vi "Sched select.vi"() -> (0 "Close":bool, 1 "Load":bool, 3 "selected sched":string)   [LabVIEW 2023]
uses:
  Sched select.ctl
panel:
  in  "stop":bool
  in  "Schedules":T1
  out "SchedNames":string[](array[string])
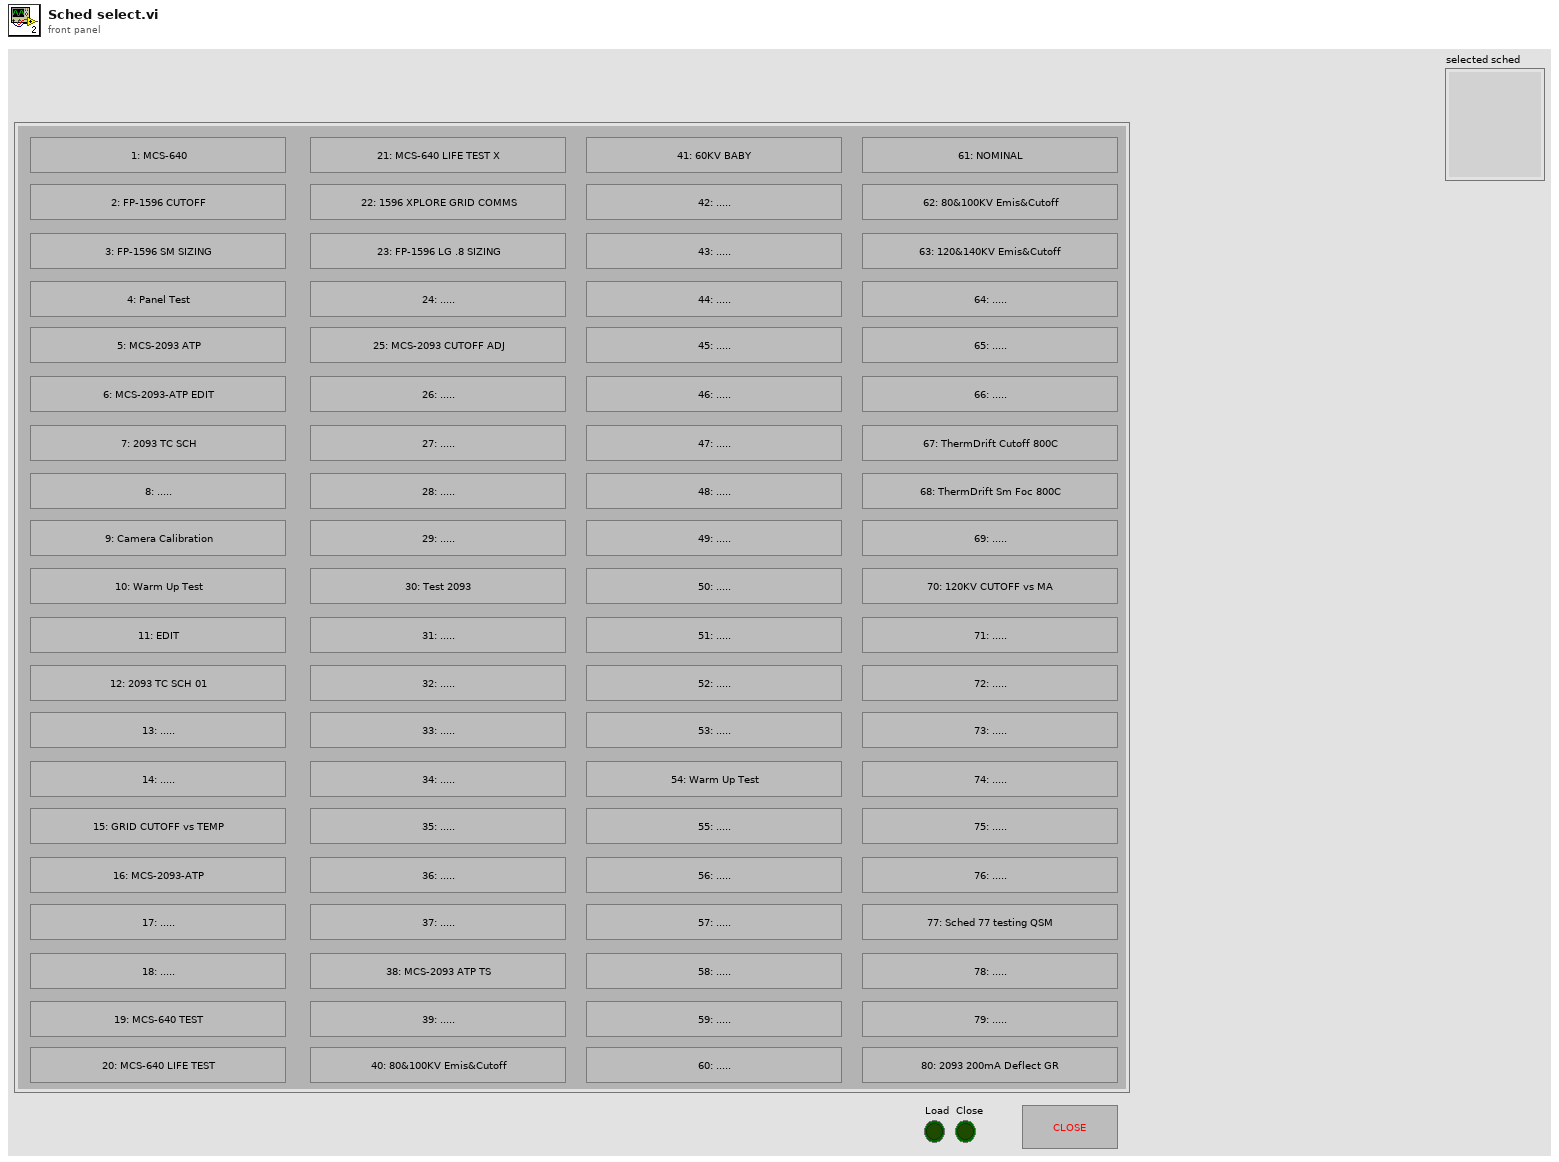
[diagram p1: front panel]
types:
  T1 = typedef "Sched select.ctl" = cluster{"OK Button 1":bool, "OK Button 2":bool, "OK Button 3":bool, "OK Button 4":bool, "OK Button 5":bool, "OK Button 6":bool, "OK Button 7":bool, "OK Button 8":bool, "OK Button 9":bool, "OK Button 10":bool, "OK Button 11":bool, "OK Button 12":bool, "OK Button 13":bool, "OK Button 14":bool, "OK Button 15":bool, "OK Button 16":bool, "OK Button 17":bool, "OK Button 18":bool, "OK Button 19":bool, "OK Button 20":bool, "OK Button 21":bool, "OK Button 22":bool, "OK Button 23":bool, "OK Button 24":bool, "OK Button 25":bool, "OK Button 26":bool, "OK Button 27":bool, "OK Button 28":bool, "OK Button 29":bool, "OK Button 30":bool, "OK Button 31":bool, "OK Button 32":bool, "OK Button 33":bool, "OK Button 34":bool, "OK Button 35":bool, "OK Button 36":bool, "OK Button 37":bool, "OK Button 38":bool, "OK Button 39":bool, "OK Button 40":bool, "OK Button 41":bool, "OK Button 42":bool, "OK Button 43":bool, "OK Button 44":bool, "OK Button 45":bool, "OK Button 46":bool, "OK Button 47":bool, "OK Button 48":bool, "OK Button 49":bool, "OK Button 50":bool, "OK Button 51":bool, "OK Button 52":bool, "OK Button 53":bool, "OK Button 54":bool, "OK Button 55":bool, "OK Button 56":bool, "OK Button 57":bool, "OK Button 58":bool, "OK Button 59":bool, "OK Button 60":bool, "OK Button 61":bool, "OK Button 62":bool, "OK Button 63":bool, "OK Button 64":bool, "OK Button 65":bool, "OK Button 66":bool, "OK Button 67":bool, "OK Button 68":bool, "OK Button 69":bool, "OK Button 70":bool, "OK Button 71":bool, "OK Button 72":bool, "OK Button 73":bool, "OK Button 74":bool, "OK Button 75":bool, "OK Button 76":bool, "OK Button 77":bool, "OK Button 78":bool, "OK Button 79":bool, "OK Button 80":bool}
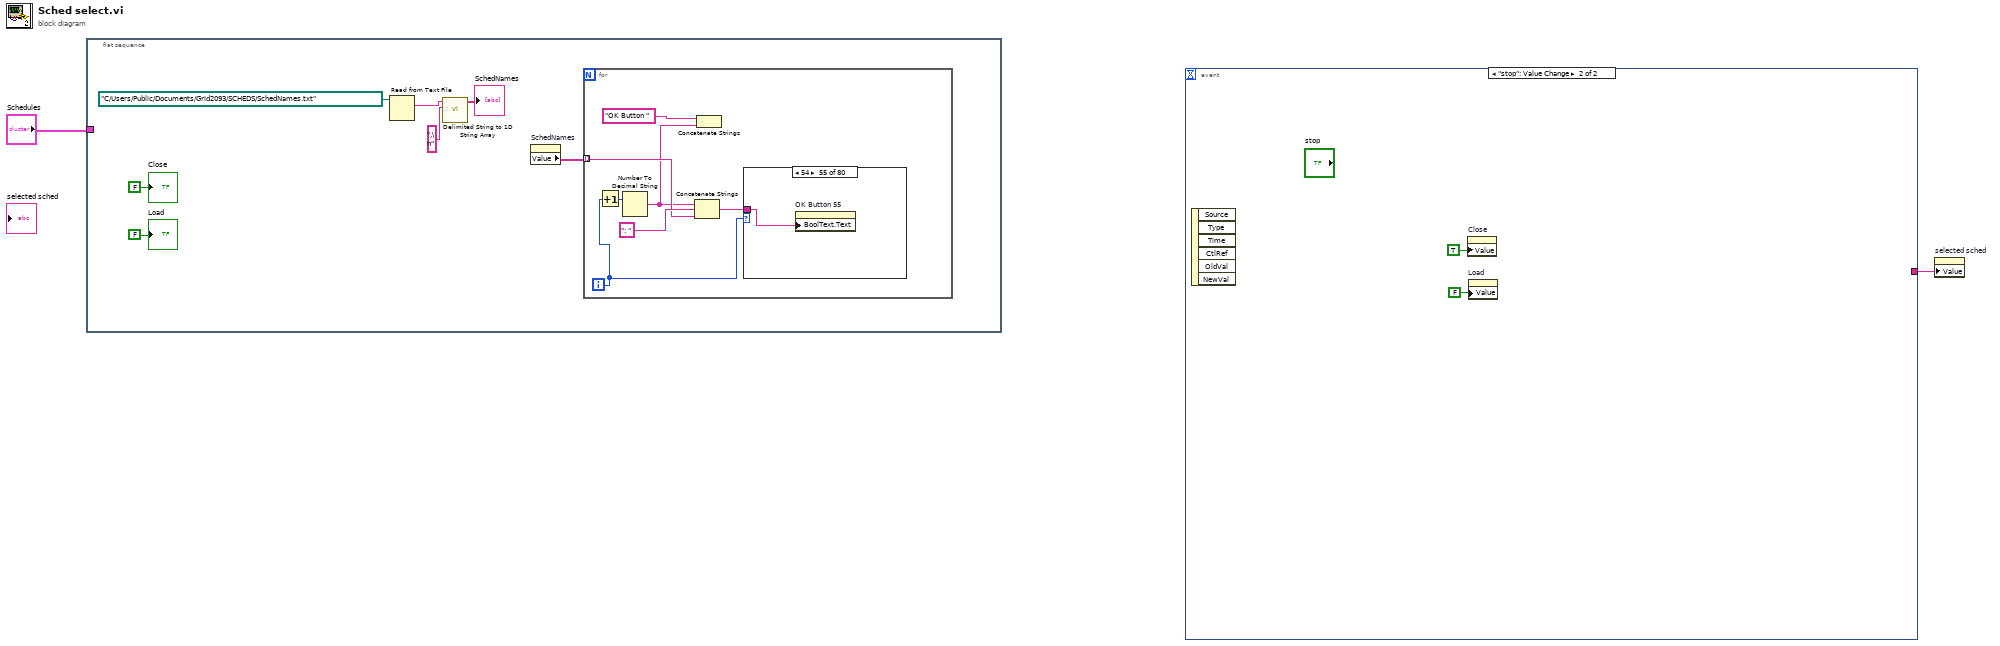
[diagram p0: block diagram]
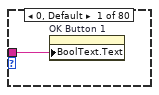
[diagram p2: hidden frame]
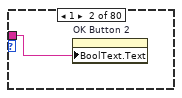
[diagram p3: hidden frame]
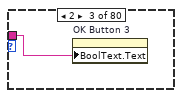
[diagram p4: hidden frame]
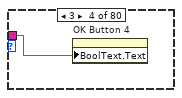
[diagram p5: hidden frame]
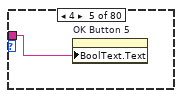
[diagram p6: hidden frame]
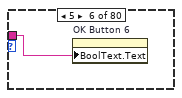
[diagram p7: hidden frame]
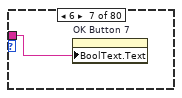
[diagram p8: hidden frame]
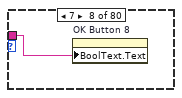
[diagram p9: hidden frame]
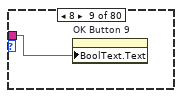
[diagram p10: hidden frame]
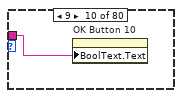
[diagram p11: hidden frame]
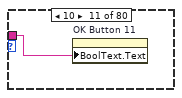
[diagram p12: hidden frame]
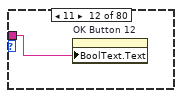
[diagram p13: hidden frame]
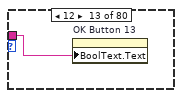
[diagram p14: hidden frame]
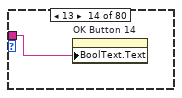
[diagram p15: hidden frame]
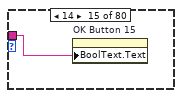
[diagram p16: hidden frame]
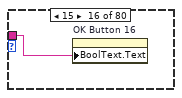
[diagram p17: hidden frame]
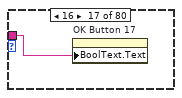
[diagram p18: hidden frame]
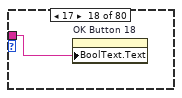
[diagram p19: hidden frame]
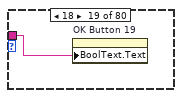
[diagram p20: hidden frame]
diagram:
  n1 = flat-sequence {
    tunnel: "Schedules" -> [_]
    frame #0 {
      n2 = Read from Text File(file (use dialog)=path "C:/Users/Public/Documents/Grid2093/SCHEDS/SchedNames.txt") -> (text=w9:string)  [unwired: 3 in, 3 out]
      n3 = call <vilib>:"Delimited String to 1D String Array.vi"("delimiter"=",\n", "delimited string"=w9) -> ("string array"=→"SchedNames":string[])  [unwired: 9 in]
      n4 = property on="SchedNames" class="Arr (strict)"() -> ("Value"=w6:string[])  [unwired: 2 in, 2 out]
      n5 = for {
        tunnel: w6 -> [w15] mode=indexing
        i -> [w11]
        n6 = Increment(x=w11) -> (x+1=w12:i32)
        n7 = Number To Decimal String(number=w12) -> (decimal integer string=w13:string)  [unwired: 1 in]
        n8 = Concatenate Strings(w13, ": " ("string"), w15) -> (w10:string)
        n9 = Concatenate Strings("OK Button ", w13) -> ()  [unwired: 1 out]
        n10 = case shown="54" w11 {
          tunnel: w10 -> [w17 w18 w19 w20 w21 w22 w23 w24 w25 w26 w27 w28 w29 w30 w31 w32 w33 w34 w35 w36 w37 w38 w39 w40 w41 w42 w43 w44 w45 w46 w47 w48 w49 w50 w51 w52 w53 w54 w55 w56 w57 w58 w59 w60 w61 w62 w63 w64 w65 w66 w67 w68 w69 w70 w71 w72 w73 w74 w75 w76 w77 w78 w79 w80 w81 w82 w83 w84 w85 w86 w87 w88 w89 w90 w91 w92 w93 w94 w95 w96]
          frame 0, Default {
            n11 = property on="OK Button 1" class="Bool (strict)"("BoolText.Text"=w17) -> ()  [unwired: 2 in, 2 out]
          }
          frame 1 {
            n12 = property on="OK Button 2" class="Bool (strict)"("BoolText.Text"=w18) -> ()  [unwired: 2 in, 2 out]
          }
          frame 2 {
            n13 = property on="OK Button 3" class="Bool (strict)"("BoolText.Text"=w19) -> ()  [unwired: 2 in, 2 out]
          }
          frame 3 {
            n14 = property on="OK Button 4" class="Bool (strict)"("BoolText.Text"=w20) -> ()  [unwired: 2 in, 2 out]
          }
          frame 4 {
            n15 = property on="OK Button 5" class="Bool (strict)"("BoolText.Text"=w21) -> ()  [unwired: 2 in, 2 out]
          }
          frame 5 {
            n16 = property on="OK Button 6" class="Bool (strict)"("BoolText.Text"=w22) -> ()  [unwired: 2 in, 2 out]
          }
          frame 6 {
            n17 = property on="OK Button 7" class="Bool (strict)"("BoolText.Text"=w23) -> ()  [unwired: 2 in, 2 out]
          }
          frame 7 {
            n18 = property on="OK Button 8" class="Bool (strict)"("BoolText.Text"=w24) -> ()  [unwired: 2 in, 2 out]
          }
          frame 8 {
            n19 = property on="OK Button 9" class="Bool (strict)"("BoolText.Text"=w25) -> ()  [unwired: 2 in, 2 out]
          }
          frame 9 {
            n20 = property on="OK Button 10" class="Bool (strict)"("BoolText.Text"=w26) -> ()  [unwired: 2 in, 2 out]
          }
          frame 10 {
            n21 = property on="OK Button 11" class="Bool (strict)"("BoolText.Text"=w27) -> ()  [unwired: 2 in, 2 out]
          }
          frame 11 {
            n22 = property on="OK Button 12" class="Bool (strict)"("BoolText.Text"=w28) -> ()  [unwired: 2 in, 2 out]
          }
          frame 12 {
            n23 = property on="OK Button 13" class="Bool (strict)"("BoolText.Text"=w29) -> ()  [unwired: 2 in, 2 out]
          }
          frame 13 {
            n24 = property on="OK Button 14" class="Bool (strict)"("BoolText.Text"=w30) -> ()  [unwired: 2 in, 2 out]
          }
          frame 14 {
            n25 = property on="OK Button 15" class="Bool (strict)"("BoolText.Text"=w31) -> ()  [unwired: 2 in, 2 out]
          }
          frame 15 {
            n26 = property on="OK Button 16" class="Bool (strict)"("BoolText.Text"=w32) -> ()  [unwired: 2 in, 2 out]
          }
          frame 16 {
            n27 = property on="OK Button 17" class="Bool (strict)"("BoolText.Text"=w33) -> ()  [unwired: 2 in, 2 out]
          }
          frame 17 {
            n28 = property on="OK Button 18" class="Bool (strict)"("BoolText.Text"=w34) -> ()  [unwired: 2 in, 2 out]
          }
          frame 18 {
            n29 = property on="OK Button 19" class="Bool (strict)"("BoolText.Text"=w35) -> ()  [unwired: 2 in, 2 out]
          }
          frame 19 {
            n30 = property on="OK Button 20" class="Bool (strict)"("BoolText.Text"=w36) -> ()  [unwired: 2 in, 2 out]
          }
          frame 20 {
            n31 = property on="OK Button 21" class="Bool (strict)"("BoolText.Text"=w37) -> ()  [unwired: 2 in, 2 out]
          }
          frame 21 {
            n32 = property on="OK Button 22" class="Bool (strict)"("BoolText.Text"=w38) -> ()  [unwired: 2 in, 2 out]
          }
          frame 22 {
            n33 = property on="OK Button 23" class="Bool (strict)"("BoolText.Text"=w39) -> ()  [unwired: 2 in, 2 out]
          }
          frame 23 {
            n34 = property on="OK Button 24" class="Bool (strict)"("BoolText.Text"=w40) -> ()  [unwired: 2 in, 2 out]
          }
          frame 24 {
            n35 = property on="OK Button 25" class="Bool (strict)"("BoolText.Text"=w41) -> ()  [unwired: 2 in, 2 out]
          }
          frame 25 {
            n36 = property on="OK Button 26" class="Bool (strict)"("BoolText.Text"=w42) -> ()  [unwired: 2 in, 2 out]
          }
          frame 26 {
            n37 = property on="OK Button 27" class="Bool (strict)"("BoolText.Text"=w43) -> ()  [unwired: 2 in, 2 out]
          }
          frame 27 {
            n38 = property on="OK Button 28" class="Bool (strict)"("BoolText.Text"=w44) -> ()  [unwired: 2 in, 2 out]
          }
          frame 28 {
            n39 = property on="OK Button 29" class="Bool (strict)"("BoolText.Text"=w45) -> ()  [unwired: 2 in, 2 out]
          }
          frame 29 {
            n40 = property on="OK Button 30" class="Bool (strict)"("BoolText.Text"=w46) -> ()  [unwired: 2 in, 2 out]
          }
          frame 30 {
            n41 = property on="OK Button 31" class="Bool (strict)"("BoolText.Text"=w47) -> ()  [unwired: 2 in, 2 out]
          }
          frame 31 {
            n42 = property on="OK Button 32" class="Bool (strict)"("BoolText.Text"=w48) -> ()  [unwired: 2 in, 2 out]
          }
          frame 32 {
            n43 = property on="OK Button 33" class="Bool (strict)"("BoolText.Text"=w49) -> ()  [unwired: 2 in, 2 out]
          }
          frame 33 {
            n44 = property on="OK Button 34" class="Bool (strict)"("BoolText.Text"=w50) -> ()  [unwired: 2 in, 2 out]
          }
          frame 34 {
            n45 = property on="OK Button 35" class="Bool (strict)"("BoolText.Text"=w51) -> ()  [unwired: 2 in, 2 out]
          }
          frame 35 {
            n46 = property on="OK Button 36" class="Bool (strict)"("BoolText.Text"=w52) -> ()  [unwired: 2 in, 2 out]
          }
          frame 36 {
            n47 = property on="OK Button 37" class="Bool (strict)"("BoolText.Text"=w53) -> ()  [unwired: 2 in, 2 out]
          }
          frame 37 {
            n48 = property on="OK Button 38" class="Bool (strict)"("BoolText.Text"=w54) -> ()  [unwired: 2 in, 2 out]
          }
          frame 38 {
            n49 = property on="OK Button 39" class="Bool (strict)"("BoolText.Text"=w55) -> ()  [unwired: 2 in, 2 out]
          }
          frame 39 {
            n50 = property on="OK Button 40" class="Bool (strict)"("BoolText.Text"=w56) -> ()  [unwired: 2 in, 2 out]
          }
          frame 40 {
            n51 = property on="OK Button 41" class="Bool (strict)"("BoolText.Text"=w57) -> ()  [unwired: 2 in, 2 out]
          }
          frame 41 {
            n52 = property on="OK Button 42" class="Bool (strict)"("BoolText.Text"=w58) -> ()  [unwired: 2 in, 2 out]
          }
          frame 42 {
            n53 = property on="OK Button 43" class="Bool (strict)"("BoolText.Text"=w59) -> ()  [unwired: 2 in, 2 out]
          }
          frame 43 {
            n54 = property on="OK Button 44" class="Bool (strict)"("BoolText.Text"=w60) -> ()  [unwired: 2 in, 2 out]
          }
          frame 44 {
            n55 = property on="OK Button 45" class="Bool (strict)"("BoolText.Text"=w61) -> ()  [unwired: 2 in, 2 out]
          }
          frame 45 {
            n56 = property on="OK Button 46" class="Bool (strict)"("BoolText.Text"=w62) -> ()  [unwired: 2 in, 2 out]
          }
          frame 46 {
            n57 = property on="OK Button 47" class="Bool (strict)"("BoolText.Text"=w63) -> ()  [unwired: 2 in, 2 out]
          }
          frame 47 {
            n58 = property on="OK Button 48" class="Bool (strict)"("BoolText.Text"=w64) -> ()  [unwired: 2 in, 2 out]
          }
          frame 48 {
            n59 = property on="OK Button 49" class="Bool (strict)"("BoolText.Text"=w65) -> ()  [unwired: 2 in, 2 out]
          }
          frame 49 {
            n60 = property on="OK Button 50" class="Bool (strict)"("BoolText.Text"=w66) -> ()  [unwired: 2 in, 2 out]
          }
          frame 50 {
            n61 = property on="OK Button 51" class="Bool (strict)"("BoolText.Text"=w67) -> ()  [unwired: 2 in, 2 out]
          }
          frame 51 {
            n62 = property on="OK Button 52" class="Bool (strict)"("BoolText.Text"=w68) -> ()  [unwired: 2 in, 2 out]
          }
          frame 52 {
            n63 = property on="OK Button 53" class="Bool (strict)"("BoolText.Text"=w69) -> ()  [unwired: 2 in, 2 out]
          }
          frame 53 {
            n64 = property on="OK Button 54" class="Bool (strict)"("BoolText.Text"=w70) -> ()  [unwired: 2 in, 2 out]
          }
          frame 54 {
            n65 = property on="OK Button 55" class="Bool (strict)"("BoolText.Text"=w71) -> ()  [unwired: 2 in, 2 out]
          }
          frame 55 {
            n66 = property on="OK Button 56" class="Bool (strict)"("BoolText.Text"=w72) -> ()  [unwired: 2 in, 2 out]
          }
          frame 56 {
            n67 = property on="OK Button 57" class="Bool (strict)"("BoolText.Text"=w73) -> ()  [unwired: 2 in, 2 out]
          }
          frame 57 {
            n68 = property on="OK Button 58" class="Bool (strict)"("BoolText.Text"=w74) -> ()  [unwired: 2 in, 2 out]
          }
          frame 58 {
            n69 = property on="OK Button 59" class="Bool (strict)"("BoolText.Text"=w75) -> ()  [unwired: 2 in, 2 out]
          }
          frame 59 {
            n70 = property on="OK Button 60" class="Bool (strict)"("BoolText.Text"=w76) -> ()  [unwired: 2 in, 2 out]
          }
          frame 60 {
            n71 = property on="OK Button 61" class="Bool (strict)"("BoolText.Text"=w77) -> ()  [unwired: 2 in, 2 out]
          }
          frame 61 {
            n72 = property on="OK Button 62" class="Bool (strict)"("BoolText.Text"=w78) -> ()  [unwired: 2 in, 2 out]
          }
          frame 62 {
            n73 = property on="OK Button 63" class="Bool (strict)"("BoolText.Text"=w79) -> ()  [unwired: 2 in, 2 out]
          }
          frame 63 {
            n74 = property on="OK Button 64" class="Bool (strict)"("BoolText.Text"=w80) -> ()  [unwired: 2 in, 2 out]
          }
          frame 64 {
            n75 = property on="OK Button 65" class="Bool (strict)"("BoolText.Text"=w81) -> ()  [unwired: 2 in, 2 out]
          }
          frame 65 {
            n76 = property on="OK Button 66" class="Bool (strict)"("BoolText.Text"=w82) -> ()  [unwired: 2 in, 2 out]
          }
          frame 66 {
            n77 = property on="OK Button 67" class="Bool (strict)"("BoolText.Text"=w83) -> ()  [unwired: 2 in, 2 out]
          }
          frame 67 {
            n78 = property on="OK Button 68" class="Bool (strict)"("BoolText.Text"=w84) -> ()  [unwired: 2 in, 2 out]
          }
          frame 68 {
            n79 = property on="OK Button 69" class="Bool (strict)"("BoolText.Text"=w85) -> ()  [unwired: 2 in, 2 out]
          }
          frame 69 {
            n80 = property on="OK Button 70" class="Bool (strict)"("BoolText.Text"=w86) -> ()  [unwired: 2 in, 2 out]
          }
          frame 70 {
            n81 = property on="OK Button 71" class="Bool (strict)"("BoolText.Text"=w87) -> ()  [unwired: 2 in, 2 out]
          }
          frame 71 {
            n82 = property on="OK Button 72" class="Bool (strict)"("BoolText.Text"=w88) -> ()  [unwired: 2 in, 2 out]
          }
          frame 72 {
            n83 = property on="OK Button 73" class="Bool (strict)"("BoolText.Text"=w89) -> ()  [unwired: 2 in, 2 out]
          }
          frame 73 {
            n84 = property on="OK Button 74" class="Bool (strict)"("BoolText.Text"=w90) -> ()  [unwired: 2 in, 2 out]
          }
          frame 74 {
            n85 = property on="OK Button 75" class="Bool (strict)"("BoolText.Text"=w91) -> ()  [unwired: 2 in, 2 out]
          }
          frame 75 {
            n86 = property on="OK Button 76" class="Bool (strict)"("BoolText.Text"=w92) -> ()  [unwired: 2 in, 2 out]
          }
          frame 76 {
            n87 = property on="OK Button 77" class="Bool (strict)"("BoolText.Text"=w93) -> ()  [unwired: 2 in, 2 out]
          }
          frame 77 {
            n88 = property on="OK Button 78" class="Bool (strict)"("BoolText.Text"=w94) -> ()  [unwired: 2 in, 2 out]
          }
          frame 78 {
            n89 = property on="OK Button 79" class="Bool (strict)"("BoolText.Text"=w95) -> ()  [unwired: 2 in, 2 out]
          }
          frame 79 {
            n90 = property on="OK Button 80" class="Bool (strict)"("BoolText.Text"=w96) -> ()  [unwired: 2 in, 2 out]
          }
        }
      }
      "Close" <- FALSE ("Close")
      "Load" <- FALSE ("Load")
    }
  }
  n91 = event shown="[1] \"stop\": Value Change" {
    selector: _ -> [_ _]
    dyn-events: _ -> [_ _]
    timeout: _ -> [_ _]
    tunnel: [w101 _] -> w2
    event Value Change {
      n92 = event-data() -> ("OldVal"=w97:T1, "NewVal"=w98:T1)  [unwired: 1 in, 4 out]
      n93 = property on="Schedules" class="Clust (strict)"("Value"=w97) -> ()  [unwired: 2 in, 2 out]
      n94 = Unbundle(w98) -> ("OK Button 1"=w103:bool, "OK Button 2"=w104:bool, "OK Button 3"=w105:bool, "OK Button 4"=w106:bool, "OK Button 5"=w107:bool, "OK Button 6"=w108:bool, "OK Button 7"=w109:bool, "OK Button 8"=w110:bool, "OK Button 9"=w111:bool, "OK Button 10"=w112:bool, "OK Button 11"=w113:bool, "OK Button 12"=w114:bool, "OK Button 13"=w115:bool, "OK Button 14"=w116:bool, "OK Button 15"=w117:bool, "OK Button 16"=w118:bool, "OK Button 17"=w119:bool, "OK Button 18"=w120:bool, "OK Button 19"=w121:bool, "OK Button 20"=w122:bool, "OK Button 21"=w123:bool, "OK Button 22"=w124:bool, "OK Button 23"=w125:bool, "OK Button 24"=w126:bool, "OK Button 25"=w127:bool, "OK Button 26"=w128:bool, "OK Button 27"=w129:bool, "OK Button 28"=w130:bool, "OK Button 29"=w131:bool, "OK Button 30"=w132:bool, "OK Button 31"=w133:bool, "OK Button 32"=w134:bool, "OK Button 33"=w135:bool, "OK Button 34"=w136:bool, "OK Button 35"=w137:bool, "OK Button 36"=w138:bool, "OK Button 37"=w139:bool, "OK Button 38"=w140:bool, "OK Button 39"=w141:bool, "OK Button 40"=w142:bool, "OK Button 41"=w143:bool, "OK Button 42"=w144:bool, "OK Button 43"=w145:bool, "OK Button 44"=w146:bool, "OK Button 45"=w147:bool, "OK Button 46"=w148:bool, "OK Button 47"=w149:bool, "OK Button 48"=w150:bool, "OK Button 49"=w151:bool, "OK Button 50"=w152:bool, "OK Button 51"=w153:bool, "OK Button 52"=w154:bool, "OK Button 53"=w155:bool, "OK Button 54"=w156:bool, "OK Button 55"=w157:bool, "OK Button 56"=w158:bool, "OK Button 57"=w159:bool, "OK Button 58"=w160:bool, "OK Button 59"=w161:bool, "OK Button 60"=w162:bool, "OK Button 61"=w163:bool, "OK Button 62"=w164:bool, "OK Button 63"=w165:bool, "OK Button 64"=w166:bool, "OK Button 65"=w167:bool, "OK Button 66"=w168:bool, "OK Button 67"=w169:bool, "OK Button 68"=w170:bool, "OK Button 69"=w171:bool, "OK Button 70"=w173:bool, "OK Button 71"=w172:bool, "OK Button 72"=w174:bool, "OK Button 73"=w176:bool, "OK Button 74"=w175:bool, "OK Button 75"=w177:bool, "OK Button 76"=w178:bool, "OK Button 77"=w179:bool, "OK Button 78"=w180:bool, "OK Button 79"=w181:bool, "OK Button 80"=w182:bool)
      n95 = Build Array(w103, w104, w105, w106, w107, w108, w109, w110, w111, w112, w113, w114, w115, w116, w117, w118, w119, w120, w121, w122, w123, w124, w125, w126, w127, w128, w129, w130, w131, w132, w133, w134, w135, w136, w137, w138, w139, w140, w141, w142, w143, w144, w145, w146, w147, w148, w149, w150, w151, w152, w153, w154, w155, w156, w157, w158, w159, w160, w161, w162, w163, w164, w165, w166, w167, w168, w169, w170, w171, w173, w172, w174, w176, w175, w177, w178, w179, w180, w181, w182) -> (w102:bool[])
      n96 = while {
        tunnel: w102 -> [w183] mode=indexing
        tunnel: [w184] -> w101
        i -> [w185]
        stop <- w183 stop-if-true
        n97 = case shown="True" w183 {
          tunnel: w185 -> [_ w187]
          tunnel: [_ w186] -> w184
          frame False {
          }
          frame True {
            n98 = Increment(x=w187) -> (x+1=w188:i32)
            n99 = Number To Decimal String(number=w188) -> (decimal integer string=w189:string)  [unwired: 1 in]
            n100 = Concatenate Strings("Sched", w189) -> (w186:string)
          }
        }
      }
      n101 = property on="Close" class="Bool (strict)"("Value"=FALSE ("Close")) -> ()  [unwired: 2 in, 2 out]
      n102 = property on="Load" class="Bool (strict)"("Value"=TRUE ("Load")) -> ()  [unwired: 2 in, 2 out]
    }
    event "stop": Value Change {
      n103 = event-data() -> ()  [unwired: 1 in, 6 out]
      n104 = property on="Close" class="Bool (strict)"("Value"=TRUE ("Close")) -> ()  [unwired: 2 in, 2 out]
      n105 = property on="Load" class="Bool (strict)"("Value"=FALSE ("Load")) -> ()  [unwired: 2 in, 2 out]
    }
  }
  n106 = property on="selected sched" class="Str"("Value"=w2) -> ()  [unwired: 2 in, 2 out]
